vi "Begin.vi"(8 "error in":errorcluster) -> (0 "error out":errorcluster)   [LabVIEW 2017]
doc: "Called before other user functions, this VI is expected to open initial I/O refnums, load in file data, and do all program initialization. Notice that the <B>error out</B> terminal is simply used for data flow. Wiring it to other structures or subVIs ensures that this VI runs first."
uses:
  <vilib>/Rock Robotics/WPI/DriverStation/WPI_DriverStationRobotMode2.ctl
  <vilib>/Rock Robotics/WPI/Joystick/WPI_JoystickDeviceEnum.ctl
  <vilib>/Rock Robotics/WPI/Solenoid/WPI_SolenoidChannel.ctl
  <vilib>/Rock Robotics/SystemInterfaces/DIO/FPGA_DIORelayChannel.ctl
  <vilib>/Rock Robotics/WPI/Solenoid/WPI_SolenoidValue.ctl
  <vilib>/Rock Robotics/WPI/ThirdParty/Phoenix-LabVIEW/Motor Controller/Controls/CTRE_Phoenix_MotorControl_FeedbackDevice.ctl
  <vilib>/Rock Robotics/WPI/ThirdParty/Phoenix-LabVIEW/Motor Controller/Controls/CTRE_Phoenix_MotorControl_NeutralMode.ctl
  <vilib>/Rock Robotics/SystemInterfaces/AI/FPGA_AIChannel.ctl
  <vilib>/Rock Robotics/SystemInterfaces/DIO/FPGA_DIOChannel.ctl
  Robot Global Data.vi
  <vilib>/Rock Robotics/Network Tables/NT Write String Array.vi
  <vilib>/Rock Robotics/WPI/RobotDrive/WPI_RobotDriveOpen2MotorWithExistingMotors.vi
  <vilib>/Rock Robotics/WPI/Solenoid/WPI_SolenoidOpenSingle.vi
  <vilib>/Rock Robotics/WPI/Utilities/WPI_GetSetVariantRefNum.vi
  <vilib>/Rock Robotics/WPI/Solenoid/WPI_SolenoidSetEnum.vi
  <vilib>/Rock Robotics/WPI/ThirdParty/Phoenix-LabVIEW/Pigeon IMU/CTRE_PigeonIMU_Open_CAN.vi
  <vilib>/Rock Robotics/WPI/Ultrasonic/WPI_SonarMB1010DigRefNum Registry Set.vi
  <vilib>/Rock Robotics/SystemInterfaces/spilib/spi_bus.ctl
  <vilib>/Rock Robotics/WPI/Gyro/WPI_GyroXRS450_SPI_Open.vi
  <vilib>/Rock Robotics/WPI/Ultrasonic/WPI_SonarMB1010DigitalOpen.vi
panel:
  out "error out 2":errorcluster
  in  "error in 2":errorcluster
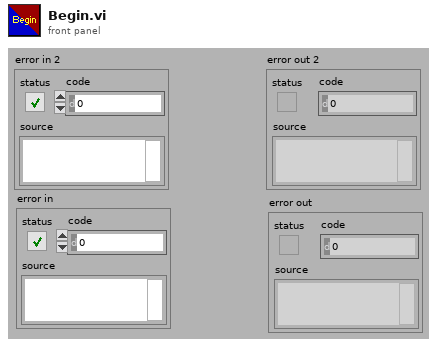
[diagram p1: front panel]
types:
  T1 = typedef "FPGA_DIOChannel.ctl" = enum8{"DIO 0", "DIO 1", "DIO 2", "DIO 3", "DIO 4", "DIO 5", "DIO 6", "DIO 7", "DIO 8", "DIO 9", "DIO MXP 0", "DIO MXP 1", "DIO MXP 2", "DIO MXP 3", "DIO MXP 4", "DIO MXP 5", "DIO MXP 6", "DIO MXP 7", "DIO MXP 8", "DIO MXP 9", "DIO MXP 10", "DIO MXP 11", "DIO MXP 12", "DIO MXP 13", "DIO MXP 14", "DIO MXP 15", "SPI Port CS1", "SPI Port CS2", "SPI Port CS3", "SPI Port MISO", "SPI Port MOSI", "Invalid"}
  T2 = typedef "FPGA_AIChannel.ctl" = enum8{"AI 0", "AI 1", "AI 2", "AI 3", "AI MXP 0", "AI MXP 1", "AI MXP 2", "AI MXP 3", "Invalid"}
  T3 = typedef "CTRE_Phoenix_MotorControl_NeutralMode.ctl" = enum8{"EEPROMSetting", "Override to Coast", "Override to Brake"}
  T4 = typedef "WPI_SolenoidValue.ctl" = enum16{"Off", "On", "Forward", "Reverse"}
  T5 = typedef "FPGA_DIORelayChannel.ctl" = enum8{"Relay 0", "Relay 1", "Relay 2", "Relay 3", "Invalid"}
  T6 = typedef "WPI_SolenoidChannel.ctl" = enum8{"Solenoid 0", "Solenoid 1", "Solenoid 2", "Solenoid 3", "Solenoid 4", "Solenoid 5", "Solenoid 6", "Solenoid 7", "Invalid"}
  T7 = typedef "WPI_JoystickDeviceEnum.ctl" = enum16{"USB 0", "USB 1", "USB 2", "USB 3", "USB 4", "USB 5"}
  T8 = typedef "WPI_DriverStationRobotMode2.ctl" = enum16{"Autonomous Disabled", "Autonomous Enabled", "Teleop Disabled", "Teleop Enabled", "Disconnected", "Finish", "Test Disabled", "Test Enabled", "Emergency Stopped"}
  T9 = typedef "spi_bus.ctl" = enum16{"SPI On-Board, CS0", "SPI On-Board, CS1", "SPI On-Board, CS2", "SPI On-Board, CS3", "SPI MXP", "Invalid"}
  T10 = typedef "CTRE_Phoenix_MotorControl_FeedbackDevice.ctl" = i8
  T11 = typedef "WPI_AnalogChannelDevRef.ctl" = cluster{"DevStatus":errorcluster, "Analog Channel":T2}
  T12 = typedef "WPI_JoystickDevRef.ctl" = cluster{"Device":T7}
  T13 = typedef "WPI_DigitalInputDevRef.ctl" = cluster{"DevStatus":errorcluster, "DIO Channel":T1}
  T14 = typedef "WPI_SolenoidDevRef.ctl" = cluster{"DevStatus":errorcluster, "Pneumatics Control Module":u8, "Forward Solenoid Channel":T6, "Reverse Solenoid Channel":T6}
  T15 = typedef "WPI_SonarMB1010DigitalDeviceRef.ctl" = cluster{"CounterDevRef":T16, "Scaling factor (s/in)":dbl}
  T16 = typedef "WPI_CounterDevRef.ctl" = cluster{"DevStatus":errorcluster, "CntIndex":T17}
  T17 = typedef "FPGA_CounterCtrSystemIndex.ctl" = enum8{"Ctr 0", "Ctr 1", "Ctr 2", "Ctr 3", "Ctr 4", "Ctr 5", "Ctr 6", "Ctr 7", "Invalid"}
  T18 = typedef "WPI_MotorControlDeviceRef.ctl" = cluster{"DeviceStatus":errorcluster, "Type":T19, "PWM":cluster{"PWM Channel":T20, "DeadBand":T21}, "CAN":cluster{"Device Number":u8, "SetOutput VI Ref":variant, "GetOutput VI Ref":variant, "Enable VI Ref":variant, "Disable VI Ref":variant, "Data":variant}, "Invert":bool, "DIO PWM":cluster{"PWM \"Enable\" Channel":T20, "DIOChannel":T1, "PWM Rate":dbl}}
  T19 = typedef "WPI_MotorControlType.ctl" = enum16{"PWM", "CAN", "DIO PWM"}
  T20 = typedef "FPGA_DIOPWMChannel.ctl" = enum8{"PWM 0", "PWM 1", "PWM 2", "PWM 3", "PWM 4", "PWM 5", "PWM 6", "PWM 7", "PWM 8", "PWM 9", "PWM MXP 0", "PWM MXP 1", "PWM MXP 2", "PWM MXP 3", "PWM MXP 4", "PWM MXP 5", "PWM MXP 6", "PWM MXP 7", "PWM MXP 8", "PWM MXP 9", "Invalid"}
  T21 = typedef "WPI_PWMDeadband.ctl" = cluster{"Name":string, "maxPositivePwm":i32, "minPositivePwm":i32, "centerPwm":i32, "maxNegativePwm":i32, "minNegativePwm":i32, "angularRange":u16}
  T22 = typedef "WPI_RelayDevRef.ctl" = cluster{"DevStatus":errorcluster, "Relay Channel":T5, "Relay Direction":T23}
  T23 = typedef "WPI_RelayDirection.ctl" = enum16{"Both directions", "Forward only", "Reverse only"}
  T24 = typedef "WPI_CompressorDevRef.ctl" = cluster{"DevStatus":errorcluster, "Pneumatics Control Module":u8}
  T25 = typedef "WPI_GyroDevRef.ctl" = cluster{"DevStatus":errorcluster, "Analog Channel":T2, "Gain (VoltsPerDegree/Second)":dbl, "Gyro Type":enum16{"Analog", "XRS450"}, "Handle":i32, "SPI Bus":T9, "Device Found":bool, "Sample Rate":dbl, "Calibrate On Open":bool, "Offset":dbl}
  T26 = typedef "CTRE_PigeonIMU_DeviceRef.ctl" = cluster{"DeviceStatus":errorcluster, "Device Number":u8, "Type":T27, "Device ID":u32, "Handle":u64, "UsageFrame":u32, "Library Path":path}
  T27 = typedef "CTRE_PigeonIMU_ConnectionType.ctl" = u32
  T28 = typedef "WPI_RobotDriveDevRef.ctl" = cluster{"DevStatus":errorcluster, "Motors[]":T18[], "Square Inputs":bool, "Max Output":dbl}
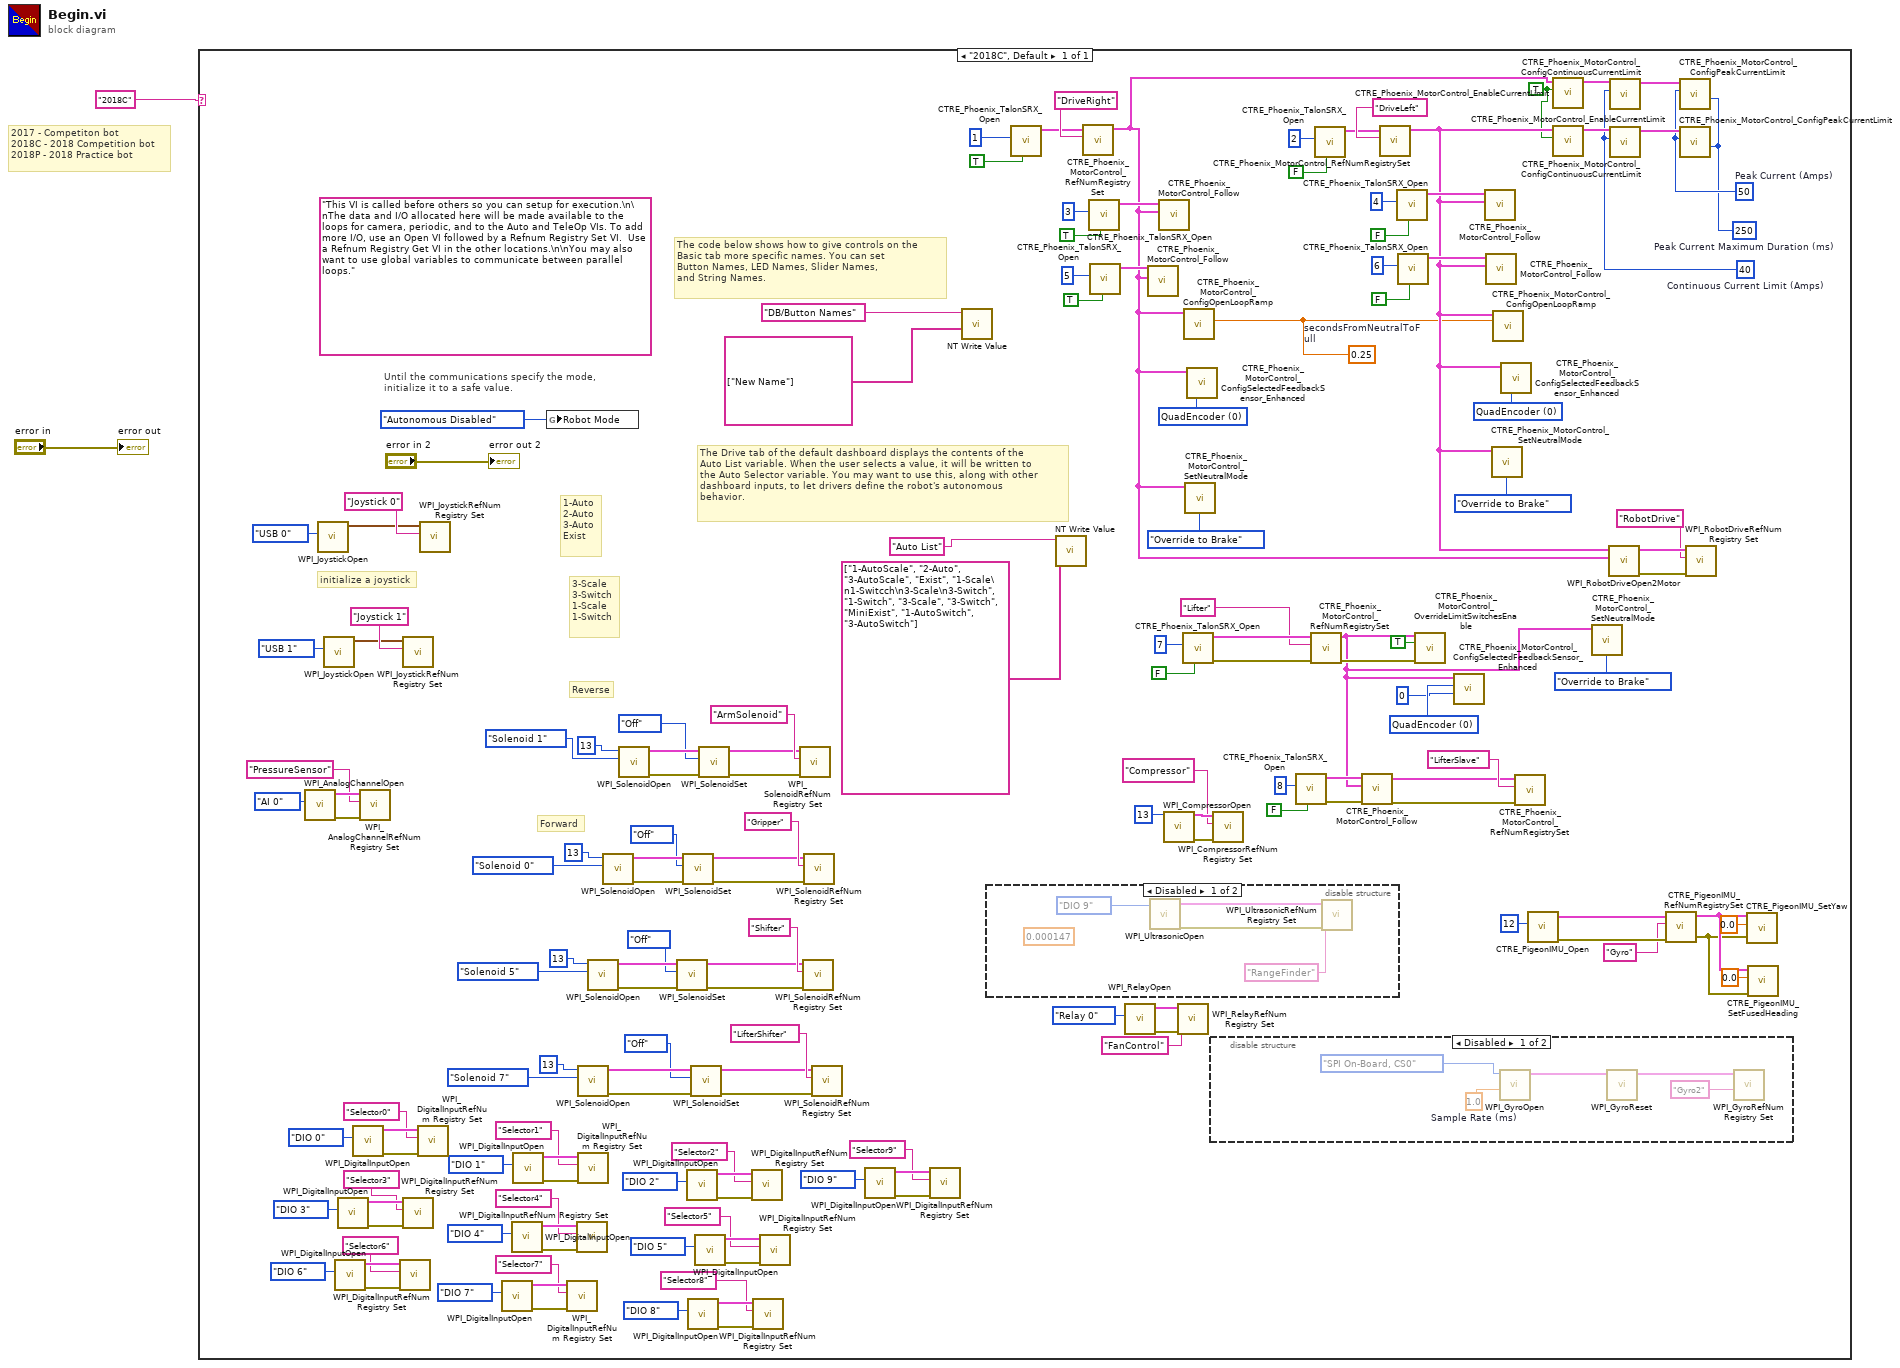
[diagram p0: block diagram]
diagram:
  # "2017 - Competiton bot\n2018C - 2018 Competition bot\n2018P - 2018 Practice bot"
  n1 = case shown="\"2018C\", Default" "2018C" {
    frame "2018C", Default {
      w53 = 250  # Peak Current Maximum Duration (ms)
      w54 = 50  # Peak Current (Amps)
      w55 = 40  # Continuous Current Limit (Amps)
      w50 = TRUE ("Enable Current Limit?")
      w69 = T10 0 items=["None"=-1, "QuadEncoder"=0, "Analog"=2, "Tachometer"=4, "Pulse Width Encoded Position"=8, "Sensor Sum (S0 + S1)"=9, "Sensor Difference (D0 - D1)"=10, "Remote Source 0"=11, "Remote Source 1"=12, "Software Emulated"=15] ("Feedback Device")
      w70 = T10 0 items=["None"=-1, "QuadEncoder"=0, "Analog"=2, "Tachometer"=4, "Pulse Width Encoded Position"=8, "Sensor Sum (S0 + S1)"=9, "Sensor Difference (D0 - D1)"=10, "Remote Source 0"=11, "Remote Source 1"=12, "Software Emulated"=15] ("Feedback Device")
      w71 = T10 0 items=["None"=-1, "QuadEncoder"=0, "Analog"=2, "Tachometer"=4, "Pulse Width Encoded Position"=8, "Sensor Sum (S0 + S1)"=9, "Sensor Difference (D0 - D1)"=10, "Remote Source 0"=11, "Remote Source 1"=12, "Software Emulated"=15] ("Feedback Device")
      w49 = 0.25  # secondsFromNeutralToFull
      (unwired) "This VI is called before others so you can setup for execution.\n\nThe data and I/O allocated here will be made available to the loops for camera, periodic, and to the Auto and TeleOp VIs. To add more I/O, use an Open VI followed by a Refnum Registry Set VI.  Use a Refnum Registry Get VI in the other locations.\n\nYou may also want to use global variables to communicate between parallel loops."
      # "1-Auto\n2-Auto\n3-Auto\nExist"
      # "3-Scale\n3-Switch\n1-Scale\n1-Switch"
      # "Forward"
      # "Reverse"
      # "The Drive tab of the default dashboard displays the contents of the\nAuto List variable. When the user selects a value, it will be written to\nthe Auto Selector variable. You may want to use this, along with other\ndashboard inputs, to let drivers define the robot's autonomous\nbehavior."
      # "The code below shows how to give controls on the\nBasic tab more specific names. You can set\nButton Names, LED Names, Slider Names,\nand String Names."
      # "initialize a joystick"
      # "Until the communications specify the mode,\ninitialize it to a safe value."
      n2 = call <vilib>:"WPI_AnalogChannelOpen.vi"("Analog Channel"=FPGA_AIChannel."AI 0") -> ("error out"=w45:errorcluster, "AIDeviceRef"=w46:T11)  [unwired: 9 in]
      n3 = call <vilib>:"WPI_JoystickOpen.vi"("JoystickDevice"=WPI_JoystickDeviceEnum."USB 0") -> ("JoystickDevRef"=w156:T12)  [unwired: 10 in]
      n4 = call <vilib>:"WPI_JoystickOpen.vi"("JoystickDevice"=WPI_JoystickDeviceEnum."USB 1") -> ("JoystickDevRef"=w112:T12)  [unwired: 10 in]
      n5 = call <vilib>:"WPI_DigitalInputOpen.vi"("DIO Channel"=FPGA_DIOChannel."DIO 6") -> ("error out"=w35:errorcluster, "DigitalInputDevRef"=w34:T13)  [unwired: 9 in]
      n6 = call <vilib>:"WPI_DigitalInputOpen.vi"("DIO Channel"=FPGA_DIOChannel."DIO 3") -> ("error out"=w38:errorcluster, "DigitalInputDevRef"=w37:T13)  [unwired: 9 in]
      n7 = call <vilib>:"WPI_DigitalInputOpen.vi"("DIO Channel"=FPGA_DIOChannel."DIO 0") -> ("error out"=w41:errorcluster, "DigitalInputDevRef"=w40:T13)  [unwired: 9 in]
      n8 = call <vilib>:"WPI_AnalogChannelRefNum Registry Set.vi"("error in (no error)"=w45, "refnum name"="PressureSensor", "AIDeviceRef"=w46) -> ()  [unwired: 7 in, 2 out]
      n9 = call <vilib>:"WPI_DigitalInputRefNum Registry Set.vi"("error in (no error)"=w35, "refnum name"="Selector6", "DigitalInputDevRef"=w34) -> ()  [unwired: 7 in, 2 out]
      n10 = call <vilib>:"WPI_JoystickRefNum Registry Set.vi"("refnum name"="Joystick 1", "JoystickDevRef"=w112) -> ()  [unwired: 8 in, 2 out]
      n11 = call <vilib>:"WPI_DigitalInputRefNum Registry Set.vi"("error in (no error)"=w38, "refnum name"="Selector3", "DigitalInputDevRef"=w37) -> ()  [unwired: 7 in, 2 out]
      n12 = call <vilib>:"WPI_DigitalInputRefNum Registry Set.vi"("error in (no error)"=w41, "refnum name"="Selector0", "DigitalInputDevRef"=w40) -> ()  [unwired: 7 in, 2 out]
      n13 = call <vilib>:"WPI_JoystickRefNum Registry Set.vi"("refnum name"="Joystick 0", "JoystickDevRef"=w156) -> ()  [unwired: 8 in, 2 out]
      n14 = call <vilib>:"WPI_DigitalInputOpen.vi"("DIO Channel"=FPGA_DIOChannel."DIO 7") -> ("error out"=w32:errorcluster, "DigitalInputDevRef"=w31:T13)  [unwired: 9 in]
      n15 = call <vilib>:"WPI_DigitalInputOpen.vi"("DIO Channel"=FPGA_DIOChannel."DIO 4") -> ("error out"=w29:errorcluster, "DigitalInputDevRef"=w28:T13)  [unwired: 9 in]
      n16 = call <vilib>:"WPI_DigitalInputOpen.vi"("DIO Channel"=FPGA_DIOChannel."DIO 1") -> ("error out"=w26:errorcluster, "DigitalInputDevRef"=w25:T13)  [unwired: 9 in]
      n17 = global write "Robot Global Data.vi" "Robot Mode"(WPI_DriverStationRobotMode2."Autonomous Disabled" ("Robot Mode")) -> ()
      n18 = call <vilib>:"WPI_DigitalInputRefNum Registry Set.vi"("error in (no error)"=w32, "refnum name"="Selector7", "DigitalInputDevRef"=w31) -> ()  [unwired: 7 in, 2 out]
      n19 = call <vilib>:"WPI_DigitalInputRefNum Registry Set.vi"("error in (no error)"=w29, "refnum name"="Selector4", "DigitalInputDevRef"=w28) -> ()  [unwired: 7 in, 2 out]
      n20 = call-poly <vilib>:"WPI_SolenoidOpen.vi"("Solenoid Channel"=WPI_SolenoidChannel."Solenoid 7" ("Forward Solenoid Channel"), "Pneumatics Control Module (0)"=u8 13) -> ("error out"=w101:errorcluster, "SolenoidDevRef"=w100:T14)  [unwired: 8 in]
      n21 = call <vilib>:"WPI_DigitalInputRefNum Registry Set.vi"("error in (no error)"=w26, "refnum name"="Selector1", "DigitalInputDevRef"=w25) -> ()  [unwired: 7 in, 2 out]
      n22 = call-poly <vilib>:"WPI_SolenoidOpen.vi"("Solenoid Channel"=WPI_SolenoidChannel."Solenoid 5" ("Forward Solenoid Channel"), "Pneumatics Control Module (0)"=u8 13) -> ("error out"=w128:errorcluster, "SolenoidDevRef"=w127:T14)  [unwired: 8 in]
      n23 = call-poly <vilib>:"WPI_SolenoidOpen.vi"("Solenoid Channel"=WPI_SolenoidChannel."Solenoid 0" ("Forward Solenoid Channel"), "Pneumatics Control Module (0)"=u8 13) -> ("error out"=w132:errorcluster, "SolenoidDevRef"=w131:T14)  [unwired: 8 in]
      n24 = call-poly <vilib>:"WPI_SolenoidOpen.vi"("Solenoid Channel"=WPI_SolenoidChannel."Solenoid 1" ("Forward Solenoid Channel"), "Pneumatics Control Module (0)"=u8 13) -> ("error out"=w136:errorcluster, "SolenoidDevRef"=w135:T14)  [unwired: 8 in]
      n25 = call-poly <vilib>:"WPI_SolenoidSet.vi"("Value"=WPI_SolenoidValue."Off", "SolenoidDevRef"=w127) -> ("SolenoidDevRef"=w77:T14)  [unwired: 8 in, 1 out]
      n26 = call-poly <vilib>:"WPI_SolenoidSet.vi"("Value"=WPI_SolenoidValue."Off", "SolenoidDevRef"=w131) -> ("SolenoidDevRef"=w81:T14)  [unwired: 8 in, 1 out]
      n27 = call <vilib>:"WPI_DigitalInputOpen.vi"("DIO Channel"=FPGA_DIOChannel."DIO 2") -> ("error out"=w23:errorcluster, "DigitalInputDevRef"=w22:T13)  [unwired: 9 in]
      n28 = call <vilib>:"WPI_DigitalInputOpen.vi"("DIO Channel"=FPGA_DIOChannel."DIO 8") -> ("error out"=w17:errorcluster, "DigitalInputDevRef"=w16:T13)  [unwired: 9 in]
      n29 = call-poly <vilib>:"WPI_SolenoidSet.vi"("Value"=WPI_SolenoidValue."Off", "SolenoidDevRef"=w100) -> ("SolenoidDevRef"=w76:T14)  [unwired: 8 in, 1 out]
      n30 = call <vilib>:"WPI_DigitalInputOpen.vi"("DIO Channel"=FPGA_DIOChannel."DIO 5") -> ("error out"=w20:errorcluster, "DigitalInputDevRef"=w19:T13)  [unwired: 9 in]
      n31 = call-poly <vilib>:"WPI_SolenoidSet.vi"("Value"=WPI_SolenoidValue."Off", "SolenoidDevRef"=w135) -> ("SolenoidDevRef"=w80:T14)  [unwired: 8 in, 1 out]
      n32 = call <vilib>:"WPI_DigitalInputRefNum Registry Set.vi"("error in (no error)"=w23, "refnum name"="Selector2", "DigitalInputDevRef"=w22) -> ()  [unwired: 7 in, 2 out]
      n33 = call <vilib>:"WPI_DigitalInputRefNum Registry Set.vi"("error in (no error)"=w17, "refnum name"="Selector8", "DigitalInputDevRef"=w16) -> ()  [unwired: 7 in, 2 out]
      n34 = call <vilib>:"WPI_DigitalInputRefNum Registry Set.vi"("error in (no error)"=w20, "refnum name"="Selector5", "DigitalInputDevRef"=w19) -> ()  [unwired: 7 in, 2 out]
      n35 = call <vilib>:"WPI_SolenoidRefNum Registry Set.vi"("error in (no error)"=w136, "refnum name"="ArmSolenoid", "SolenoidDevRef"=w80) -> ()  [unwired: 7 in, 2 out]
      n36 = call <vilib>:"WPI_SolenoidRefNum Registry Set.vi"("error in (no error)"=w128, "refnum name"="Shifter", "SolenoidDevRef"=w77) -> ()  [unwired: 7 in, 2 out]
      n37 = call <vilib>:"WPI_SolenoidRefNum Registry Set.vi"("error in (no error)"=w132, "refnum name"="Gripper", "SolenoidDevRef"=w81) -> ()  [unwired: 7 in, 2 out]
      n38 = call <vilib>:"WPI_SolenoidRefNum Registry Set.vi"("error in (no error)"=w101, "refnum name"="LifterShifter", "SolenoidDevRef"=w76) -> ()  [unwired: 7 in, 2 out]
      n39 = call <vilib>:"WPI_DigitalInputOpen.vi"("DIO Channel"=FPGA_DIOChannel."DIO 9") -> ("error out"=w5:errorcluster, "DigitalInputDevRef"=w4:T13)  [unwired: 9 in]
      n40 = call <vilib>:"WPI_DigitalInputRefNum Registry Set.vi"("error in (no error)"=w5, "refnum name"="Selector9", "DigitalInputDevRef"=w4) -> ()  [unwired: 7 in, 2 out]
      n41 = call-poly <vilib>:"NT Write Value.vi"("String Array"=string[] ["New Name"], "Name"="DB/Button Names") -> ()  [unwired: 9 in, 1 out]
      n42 = disable-structure shown="Disabled" {
        frame Disabled {
          (unwired) 0.000147 ("Scaling factor (s/in)")
          n43 = call-poly <vilib>:"WPI_UltrasonicOpen.vi"("DIO Channel"=FPGA_DIOChannel."DIO 9") -> ("error out"=w160:errorcluster, "SonarMB1010DigitalDevRef"=w161:T15)  [unwired: 9 in]
          n44 = call-poly <vilib>:"WPI_UltrasonicRefNum Registry Set.vi"("error in (no error)"=w160, "refnum name"="RangeFinder", "SonarMB1010DigitalDevRef"=w161) -> ()  [unwired: 7 in, 2 out]
        }
        frame Enabled {
        }
      }
      n45 = call <vilib>:"CTRE_Phoenix_TalonSRX_Open.vi"("Invert"=TRUE, "Device Number"=u8 1) -> ("CAN Talon SRX Ref"=w73:T18)  [unwired: 8 in, 1 out]
      n46 = call-poly <vilib>:"NT Write Value.vi"("String Array"=string[] ["1-AutoScale", "2-Auto", "3-AutoScale", "Exist", "1-Scale\n1-Switcch\n3-Scale\n3-Switch", "1-Switch", "3-Scale", "3-Switch", "MiniExist", "1-AutoSwitch", "3-AutoSwitch"], "Name"="Auto List") -> ()  [unwired: 9 in, 1 out]
      n47 = call <vilib>:"CTRE_Phoenix_MotorControl_RefNumRegistrySet.vi"("refnum name"="DriveRight", "PhoenixMotorControlDevRef"=w73) -> ("PhoenixMotorControlDevRef"=w52:T18)  [unwired: 8 in, 1 out]
      n48 = call <vilib>:"CTRE_Phoenix_TalonSRX_Open.vi"("Invert"=TRUE, "Device Number"=u8 3) -> ("CAN Talon SRX Ref"=w114:T18)  [unwired: 8 in, 1 out]
      n49 = call <vilib>:"CTRE_Phoenix_TalonSRX_Open.vi"("Invert"=TRUE, "Device Number"=u8 5) -> ("CAN Talon SRX Ref"=w95:T18)  [unwired: 8 in, 1 out]
      n50 = call <vilib>:"WPI_RelayOpen.vi"("Relay Channel"=FPGA_DIORelayChannel."Relay 0") -> ("error out"=w86:errorcluster, "RelayDevRef"=w85:T22)  [unwired: 9 in]
      n51 = call <vilib>:"CTRE_Phoenix_MotorControl_Follow.vi"("Master Controller to Follow"=w52, "PhoenixMotorControlDevRef"=w95) -> ()  [unwired: 8 in, 2 out]
      n52 = call <vilib>:"CTRE_Phoenix_MotorControl_Follow.vi"("Master Controller to Follow"=w52, "PhoenixMotorControlDevRef"=w114) -> ()  [unwired: 8 in, 2 out]
      n53 = call <vilib>:"WPI_CompressorOpen.vi"("Pneumatics Control Module (0)"=u8 13) -> ("CompressorDevRef"=w119:T24, "error out"=w120:errorcluster)  [unwired: 13 in]
      n54 = call <vilib>:"WPI_RelayRefNum Registry Set.vi"("error in (no error)"=w86, "refnum name"="FanControl", "RelayDevRef"=w85) -> ()  [unwired: 7 in, 2 out]
      n55 = call <vilib>:"CTRE_Phoenix_TalonSRX_Open.vi"("Invert"=FALSE, "Device Number"=u8 7) -> ("error out"=w110:errorcluster, "CAN Talon SRX Ref"=w109:T18)  [unwired: 8 in]
      n56 = call <vilib>:"CTRE_Phoenix_MotorControl_ConfigOpenLoopRamp.vi"("secondsFromNeutralToFull"=w49, "PhoenixMotorControlDevRef"=w52) -> ()  [unwired: 8 in, 2 out]
      n57 = call <vilib>:"CTRE_Phoenix_MotorControl_SetNeutralMode.vi"("Motor Control Neutral Mode"=CTRE_Phoenix_MotorControl_NeutralMode."Override to Brake", "PhoenixMotorControlDevRef"=w52) -> ()  [unwired: 8 in, 2 out]
      n58 = call <vilib>:"CTRE_Phoenix_MotorControl_ConfigSelectedFeedbackSensor_Enhanced.vi"("Feedback Device"=w71, "PhoenixMotorControlDevRef"=w52) -> ()  [unwired: 8 in, 2 out]
      n59 = disable-structure shown="Disabled" {
        frame Disabled {
          w164 = 1.0  # Sample Rate (ms)
          n60 = call-poly <vilib>:"WPI_GyroOpen.vi"("Sample Rate (Hz)"=w164, "SPI Bus"=spi_bus."SPI On-Board, CS0") -> ("GyroDevRef"=w166:T25)  [unwired: 7 in, 2 out]
          n61 = call <vilib>:"WPI_GyroReset.vi"("GyroDevRef"=w166) -> ("GyroDevRef"=w165:T25)  [unwired: 9 in, 1 out]
          n62 = call <vilib>:"WPI_GyroRefNum Registry Set.vi"("refnum name"="Gyro2", "GyroDevRef"=w165) -> ()  [unwired: 8 in, 2 out]
        }
        frame Enabled {
        }
      }
      n63 = call <vilib>:"WPI_CompressorRefNum Registry Set.vi"("error in (no error)"=w120, "refnum name"="Compressor", "CompressorDevRef"=w119) -> ()  [unwired: 7 in, 2 out]
      n64 = call <vilib>:"CTRE_Phoenix_TalonSRX_Open.vi"("Invert"=FALSE, "Device Number"=u8 8) -> ("error out"=w105:errorcluster, "CAN Talon SRX Ref"=w104:T18)  [unwired: 8 in]
      n65 = call <vilib>:"CTRE_Phoenix_MotorControl_RefNumRegistrySet.vi"("error in (no error)"=w110, "refnum name"="Lifter", "PhoenixMotorControlDevRef"=w109) -> ("error out"=w87:errorcluster, "PhoenixMotorControlDevRef"=w64:T18)  [unwired: 7 in]
      n66 = call <vilib>:"CTRE_Phoenix_TalonSRX_Open.vi"("Invert"=FALSE, "Device Number"=u8 2) -> ("CAN Talon SRX Ref"=w72:T18)  [unwired: 8 in, 1 out]
      n67 = call <vilib>:"CTRE_Phoenix_MotorControl_Follow.vi"("error in (no error)"=w105, "Master Controller to Follow"=w64, "PhoenixMotorControlDevRef"=w104) -> ("error out"=w91:errorcluster, "PhoenixMotorControlDevRef"=w89:T18)  [unwired: 7 in]
      n68 = call <vilib>:"CTRE_Phoenix_MotorControl_RefNumRegistrySet.vi"("refnum name"="DriveLeft", "PhoenixMotorControlDevRef"=w72) -> ("PhoenixMotorControlDevRef"=w51:T18)  [unwired: 8 in, 1 out]
      n69 = call <vilib>:"CTRE_Phoenix_TalonSRX_Open.vi"("Invert"=FALSE, "Device Number"=u8 4) -> ("CAN Talon SRX Ref"=w92:T18)  [unwired: 8 in, 1 out]
      n70 = call <vilib>:"CTRE_Phoenix_TalonSRX_Open.vi"("Invert"=FALSE, "Device Number"=u8 6) -> ("CAN Talon SRX Ref"=w137:T18)  [unwired: 8 in, 1 out]
      n71 = call <vilib>:"CTRE_Phoenix_MotorControl_OverrideLimitSwitchesEnable.vi"("PhoenixMotorControlDevRef"=w64, "Override Limit Switch Enable?"=TRUE, "error in (no error)"=w87) -> ()  [unwired: 11 in, 2 out]
      n72 = call <vilib>:"CTRE_Phoenix_MotorControl_ConfigSelectedFeedbackSensor_Enhanced.vi"("pidLoopIdx"=0, "Feedback Device"=w69, "PhoenixMotorControlDevRef"=w64) -> ()  [unwired: 7 in, 2 out]
      n73 = call <vilib>:"CTRE_Phoenix_MotorControl_Follow.vi"("Master Controller to Follow"=w51, "PhoenixMotorControlDevRef"=w92) -> ()  [unwired: 8 in, 2 out]
      n74 = call <vilib>:"CTRE_Phoenix_MotorControl_Follow.vi"("Master Controller to Follow"=w51, "PhoenixMotorControlDevRef"=w137) -> ()  [unwired: 8 in, 2 out]
      n75 = call <vilib>:"CTRE_Phoenix_MotorControl_SetNeutralMode.vi"("Motor Control Neutral Mode"=CTRE_Phoenix_MotorControl_NeutralMode."Override to Brake", "PhoenixMotorControlDevRef"=w51) -> ()  [unwired: 8 in, 2 out]
      n76 = call <vilib>:"CTRE_Phoenix_MotorControl_ConfigOpenLoopRamp.vi"("secondsFromNeutralToFull"=w49, "PhoenixMotorControlDevRef"=w51) -> ()  [unwired: 8 in, 2 out]
      n77 = call <vilib>:"CTRE_Phoenix_MotorControl_ConfigSelectedFeedbackSensor_Enhanced.vi"("Feedback Device"=w70, "PhoenixMotorControlDevRef"=w51) -> ()  [unwired: 8 in, 2 out]
      n78 = call <vilib>:"CTRE_Phoenix_MotorControl_RefNumRegistrySet.vi"("error in (no error)"=w91, "refnum name"="LifterSlave", "PhoenixMotorControlDevRef"=w89) -> ()  [unwired: 7 in, 2 out]
      n79 = call-poly <vilib>:"CTRE_PigeonIMU_Open.vi"("Device Number"=u8 12) -> ("error out"=w117:errorcluster, "PigeonIMUDevRef"=w116:T26)  [unwired: 9 in]
      n80 = call <vilib>:"CTRE_Phoenix_MotorControl_EnableCurrentLimit.vi"("Enable Current Limit?"=w50, "PhoenixMotorControlDevRef"=w52) -> ("PhoenixMotorControlDevRef"=w59:T18)  [unwired: 8 in, 1 out]
      n81 = call <vilib>:"CTRE_Phoenix_MotorControl_EnableCurrentLimit.vi"("Enable Current Limit?"=w50, "PhoenixMotorControlDevRef"=w51) -> ("PhoenixMotorControlDevRef"=w57:T18)  [unwired: 8 in, 1 out]
      n82 = call <vilib>:"CTRE_Phoenix_MotorControl_SetNeutralMode.vi"("Motor Control Neutral Mode"=CTRE_Phoenix_MotorControl_NeutralMode."Override to Brake", "PhoenixMotorControlDevRef"=w64) -> ()  [unwired: 8 in, 2 out]
      n83 = call-poly <vilib>:"WPI_RobotDriveOpen2Motor.vi"("Right Motor Dev Ref"=w52, "Left Motor Dev Ref"=w51) -> ("error out"=w144:errorcluster, "RobotDriveDevRef"=w143:T28)  [unwired: 8 in]
      n84 = call <vilib>:"CTRE_Phoenix_MotorControl_ConfigContinuousCurrentLimit.vi"("Continuous Current Limit (Amps)"=w55, "PhoenixMotorControlDevRef"=w59) -> ("PhoenixMotorControlDevRef"=w58:T18)  [unwired: 8 in, 1 out]
      n85 = call <vilib>:"CTRE_Phoenix_MotorControl_ConfigContinuousCurrentLimit.vi"("Continuous Current Limit (Amps)"=w55, "PhoenixMotorControlDevRef"=w57) -> ("PhoenixMotorControlDevRef"=w56:T18)  [unwired: 8 in, 1 out]
      n86 = call <vilib>:"CTRE_PigeonIMU_RefNumRegistrySet.vi"("error in (no error)"=w117, "refnum name"="Gyro", "PigeonIMUDevRef"=w116) -> ("error out"=w62:errorcluster, "PigeonIMUDevRef"=w63:T26)  [unwired: 7 in]
      n87 = call <vilib>:"CTRE_Phoenix_MotorControl_ConfigPeakCurrentLimit.vi"("Peak Current Maximum Duration (ms)"=w53, "Peak Current (Amps)"=w54, "PhoenixMotorControlDevRef"=w58) -> ()  [unwired: 7 in, 2 out]
      n88 = call <vilib>:"CTRE_Phoenix_MotorControl_ConfigPeakCurrentLimit.vi"("Peak Current Maximum Duration (ms)"=w53, "Peak Current (Amps)"=w54, "PhoenixMotorControlDevRef"=w56) -> ()  [unwired: 7 in, 2 out]
      n89 = call <vilib>:"WPI_RobotDriveRefNum Registry Set.vi"("error in (no error)"=w144, "refnum name"="RobotDrive", "RobotDriveDevRef"=w143) -> ()  [unwired: 7 in, 2 out]
      n90 = call <vilib>:"CTRE_PigeonIMU_SetYaw.vi"("error in (no error)"=w62, "Value"=0.0, "PigeonIMUDevRef"=w63) -> ()  [unwired: 7 in, 2 out]
      n91 = call <vilib>:"CTRE_PigeonIMU_SetFusedHeading.vi"("error in (no error)"=w62, "Value"=0.0, "PigeonIMUDevRef 2"=w63) -> ()  [unwired: 7 in, 2 out]
      "error out 2" <- "error in 2"
    }
  }
  "error out" <- "error in"
